vi "Start.vi"(9 "Team In":refnum<class "Team.lvclass">, 11 "Square in":refnum<class "Square.lvclass">) -> (1 "Team":refnum<class "Team.lvclass">, 3 "Square out":refnum<class "Square.lvclass">)   [LabVIEW 2020, in "SquareBattle.lvlib" / "Square.lvclass"]
uses:
  Square.lvclass
  Team/Team.lvclass
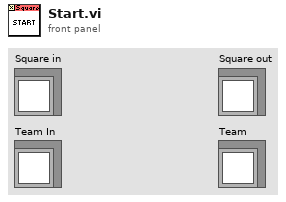
[diagram p1: front panel]
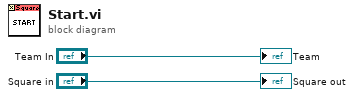
[diagram p0: block diagram]
diagram:
  "Square out" <- "Square in"
  "Team" <- "Team In"
